vi "LoadPlugin.vi"(8 "ErrorIn Array":errorcluster[](array[cluster]), 9 "PluginSelection Changed?":bool) -> (0 "ErrorOut Array":errorcluster[](array[cluster]))   [LabVIEW 2018]
doc: "This VI sends a message to load the plugin into the module."
uses:
  Queue/Queue.lvlib
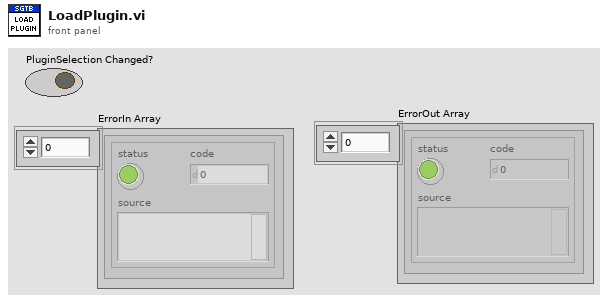
[diagram p1: front panel]
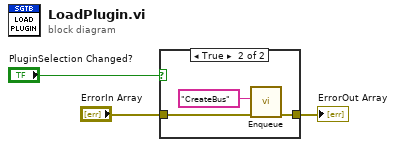
[diagram p0: block diagram]
diagram:
  n1 = case shown="True" "PluginSelection Changed?" {
    tunnel: "ErrorIn Array" -> [w4 w7]
    tunnel: [w4 w6] -> w2
    frame False {
    }
    frame True {
      n2 = call "Enqueue.vi"("ErrorArray"=w7, "Message"="CreateBus") -> ("ErrorArray"=w6:errorcluster[])  [unwired: 9 in]
    }
  }
  "ErrorOut Array" <- w2
